vi "ni579x Configure LO Enable.vi"(0 "Register Bus":T1, 1 "scope":string(combo)="LO1", 5 "enable?":bool=TRUE, 7 "wait for enable completion?":bool=TRUE, 11 "Error In":errorcluster) -> (4 "Register Bus (out)":T1, 15 "Error Out":errorcluster)   [LabVIEW 2015, in "ni579x Config v2 Host.lvlib"]
uses:
  <instrlib>/ni579x/Config/v2/Host/ni579x Config v2 Host.lvlib
  <instrlib>/_niInstr/Register Bus/v0/Host/Public/Register Bus Session.ctl
  <instrlib>/_niInstr/Register Bus/v0/Host/Private/Session Data.ctl
  <instrlib>/_niInstr/Register Bus/v0/Host/niInstr Register Bus v0 Host.lvlib
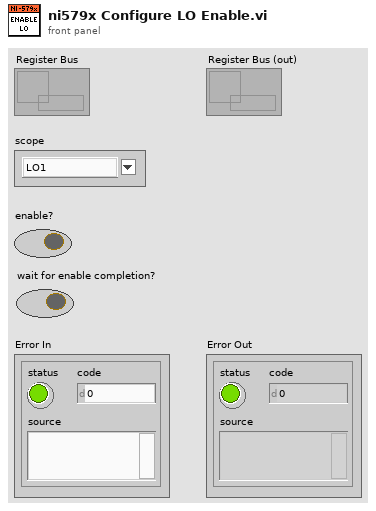
[diagram p1: front panel]
types:
  T1 = typedef "niInstr Register Bus v0 Host.lvlib/Register Bus Session.ctl" = refnum<queue>
  T2 = typedef "ni579x Config v2 Shared.lvlib/ni579x User Command.ctl" = cluster{"User Data 0":u8, "User Data 1":u8, "User Command ID":T3}
  T3 = typedef "ni579x Config v2 Shared.lvlib/ni579x User Command ID.ctl" = u8
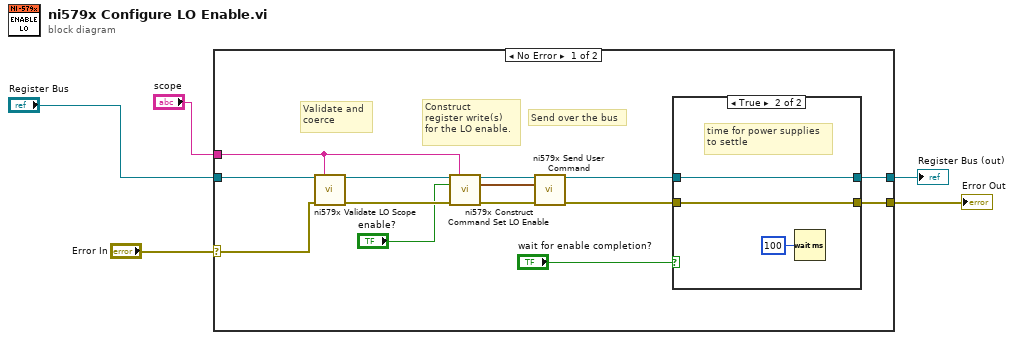
[diagram p0: block diagram]
diagram:
  n1 = case shown="No Error" "Error In" {
    selector: "Error In" -> [w18 w26]
    tunnel: [w6 w26] -> w4
    tunnel: "Register Bus" -> [w19 w25]
    tunnel: [w7 w25] -> w2
    tunnel: "scope" -> [w15 _]
    frame No Error {
      # "Construct\nregister write(s)\nfor the LO enable."
      # "Send over the bus"
      # "Validate and \ncoerce"
      n2 = call <instrlib>:"ni579x Validate LO Scope.vi"("Register Bus"=w19, "scope"=w15, "Error In"=w18) -> ("Register Bus (out)"=w17:T1, "Error Out"=w16:errorcluster)  [unwired: 11 in]
      n3 = call <instrlib>:"ni579x Construct Command Set LO Enable.vi"("Register Bus"=w17, "scope"=w15, "enable?"="enable?", "Error In"=w16) -> ("Register Bus (out)"=w14:T1, "User Command"=w13:T2, "Error Out"=w12:errorcluster)  [unwired: 9 in]
      n4 = call <instrlib>:"ni579x Send User Command.vi"("Register Bus"=w14, "User Command"=w13, "Error In"=w12) -> ("Register Bus (out)"=w9:T1, "Error Out"=w8:errorcluster)  [unwired: 8 in, 3 out]
      n5 = case shown="True" "wait for enable completion?" {
        tunnel: w9 -> [w21 w23]
        tunnel: w8 -> [w20 w22]
        tunnel: [w21 w23] -> w7
        tunnel: [w20 w22] -> w6
        frame False {
        }
        frame True {
          # "time for power supplies\nto settle"
          n6 = Wait (ms)(milliseconds to wait=u32 100) -> ()  [unwired: 1 out]
        }
      }
    }
    frame Error {
    }
  }
  "Register Bus (out)" <- w2
  "Error Out" <- w4
